vi "获取扫描电压.vi"(11 "数据":T1[](array[typedef])) -> (2 "负":dbl[](array[numeric]), 3 "正":dbl[](array[numeric]))   [LabVIEW 2020]
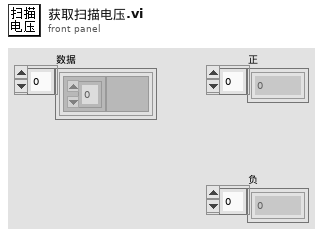
[diagram p1: front panel]
types:
  T1 = typedef "数据显示.xctl/波形数据定义.ctl" = cluster{"波形":dbl[][], "属性":variant}
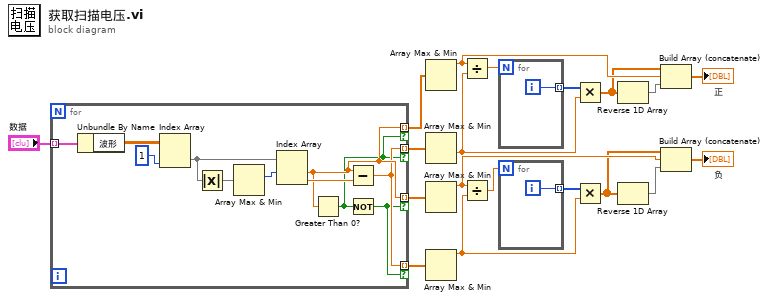
[diagram p0: block diagram]
diagram:
  n1 = for {
    tunnel: "数据" -> [w30] mode=indexing
    tunnel: [w23] -> w13 mode=indexing if=w21
    tunnel: [w22] -> w14 mode=indexing if=w21
    tunnel: [w23] -> w15 mode=indexing if=w20
    tunnel: [w22] -> w16 mode=indexing if=w20
    n2 = Unbundle By Name(w30) -> ("波形"=w27:dbl[][])
    n3 = Index Array(array=w27, index (col)=1 ("禁用的索引 (列)")) -> (element=w26:dbl[])  [unwired: 1 in]
    n4 = Absolute Value(x=w26) -> (abs(x)=w29:dbl[])
    n5 = Array Max & Min(array=w29) -> (max index (indices)=w28:i32)  [unwired: 3 out]
    n6 = Index Array(array=w26, index #1=w28) -> (element #1=w23:dbl, element #2=w24:dbl)  [unwired: 1 in]
    n7 = Greater Than 0?(x=w23) -> (x > 0?=w21:bool)
    n8 = Subtract(x=w23, y=w24) -> (x-y=w22:dbl)
    n9 = Not(x=w21) -> (.not. x?=w20:bool)
  }
  n10 = Array Max & Min(array=w13) -> (max value=w12:dbl)  [unwired: 3 out]
  n11 = Array Max & Min(array=w14) -> (min value=w3:dbl)  [unwired: 3 out]
  n12 = Array Max & Min(array=w15) -> (max value=w9:dbl)  [unwired: 3 out]
  n13 = Array Max & Min(array=w16) -> (max value=w1:dbl)  [unwired: 3 out]
  n14 = Divide(x=w12, y=w3) -> (x/y=w5:dbl)
  n15 = Divide(x=w9, y=w1) -> (x/y=w6:dbl)
  n16 = for {
    N: w5 -> [_]
    tunnel: [w31] -> w2 mode=indexing
    i -> [w31]
  }
  n17 = for {
    N: w6 -> [_]
    tunnel: [w32] -> w4 mode=indexing
    i -> [w32]
  }
  n18 = Multiply(x=w2, y=w3) -> (x*y=w11:dbl[])
  n19 = Multiply(x=w4, y=w1) -> (x*y=w7:dbl[])
  n20 = Reverse 1D Array(array=w11) -> (reversed array=w10:dbl[])
  n21 = Reverse 1D Array(array=w7) -> (reversed array=w8:dbl[])
  n22 = Build Array (concatenate)(w11, w12, w10) -> (→"正":dbl[])
  n23 = Build Array (concatenate)(w7, w9, w8) -> (→"负":dbl[])
